vi "EnQueue Action.vi"(0 "action queue in":refnum<queue>, 5 "action":string, 7 "data in":string, 9 "timeout in ms (0)":i32, 11 "error in":errorcluster, 12 "priority?":bool) -> (4 "action queue out":refnum<queue>, 15 "error out":errorcluster)   [LabVIEW 2026, in "Synchronize AWS S3 Content.lvlib" / "Actions.lvlib"]
doc: "Adds an element to the action queue.\n\n<B>Input Parameters</B>\n\n<B>action queue in</B> is a reference to a queue. Use the Create Action Queue function to obtain a queue reference. \n\n<B>action</B> inserted into system.\n\n<B>data in</B> playload into system.\n\n<B>priority element</B> set priority of action in queue.\n\n<B>timeout (ms)</B> timeout for system action.\n\n<B>error in</B> describes error conditions that occur before this node runs. This input provides standard error in functionality.\n\n<B>Output Parameters</B>\n\n<B>action queue out</B> returns the reference to the queue unchanged. \n\n<B>error out</B> contains error information. This output provides standard error out functionality."
uses:
  Actions.lvlib
  System Action Element.ctl
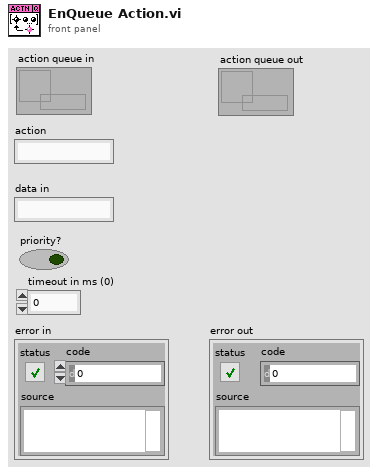
[diagram p1: front panel]
types:
  T1 = typedef "Synchronize AWS S3 Content.lvlib/Actions.lvlib/System Action Element.ctl" = cluster{"action":string, "data":string}
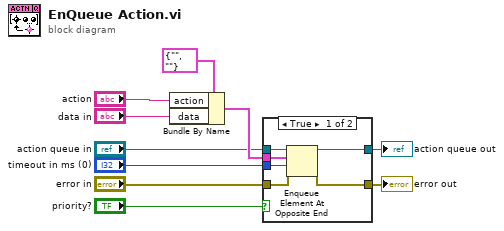
[diagram p0: block diagram]
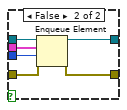
[diagram p2: hidden frame]
diagram:
  n1 = Bundle By Name(cluster=T1 {"action"="", "data"=""} ("System Action Element"), "action"="action", "data"="data in") -> (w7:T1)
  n2 = case shown="True" "priority?" {
    tunnel: "error in" -> [w13 w22]
    tunnel: [w14 w21] -> w9
    tunnel: w7 -> [w12 w20]
    tunnel: "action queue in" -> [w16 w19]
    tunnel: [w15 w18] -> w3
    tunnel: "timeout in ms (0)" -> [w11 w17]
    frame True {
      n3 = Enqueue Element At Opposite End(queue=w16, element=w12, timeout in ms (-1)=w11, error in (no error)=w13) -> (queue out=w15:refnum<queue>, error out=w14:errorcluster)  [unwired: 1 out]
    }
    frame False {
      n4 = Enqueue Element(queue=w19, element=w20, timeout in ms (-1)=w17, error in (no error)=w22) -> (queue out=w18:refnum<queue>, error out=w21:errorcluster)  [unwired: 1 out]
    }
  }
  "error out" <- w9
  "action queue out" <- w3
